vi "Locate Template.vi"(10 "Old excel":bool, 11 "File name":string) -> (3 "Path":path)   [LabVIEW 2013, in "main.lvlib"]
uses:
  main.lvlib
  Globals/DataPathGlobalVariable.vi
  <userlib>/_OpenG.lib/file/file.llb/File Exists - Scalar__ogtk.vi
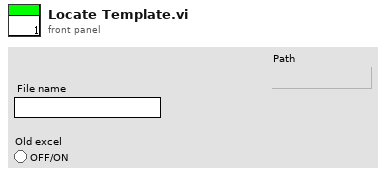
[diagram p1: front panel]
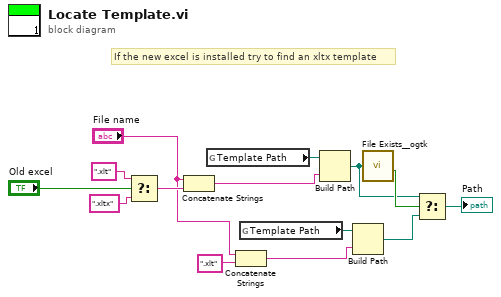
[diagram p0: block diagram]
diagram:
  # "If the new excel is installed try to find an xltx template"
  n1 = Select(t=".xlt", s="Old excel", f=".xltx") -> (s? t:f=w12:string)
  n2 = Concatenate Strings("File name", w12) -> (w9:string)
  n3 = global read "DataPathGlobalVariable.vi" "Template Path"() -> (w10:path)
  n4 = Concatenate Strings("File name", ".xlt") -> (w3:string)
  n5 = global read "DataPathGlobalVariable.vi" "Template Path"() -> (w4:path)
  n6 = Build Path(base path=w10, name or relative path=w9) -> (appended path=w5:path)
  n7 = Build Path(base path=w4, name or relative path=w3) -> (appended path=w2:path)
  n8 = call-poly <userlib>:"File Exists__ogtk.vi"("file path"=w5) -> ("exists"=w6:bool)  [unwired: 6 in, 1 out]
  n9 = Select(t=w5, s=w6, f=w2) -> (s? t:f=→"Path":path)
